vi "Thermistor Example.vi"() -> ()   [LabVIEW 2012]
doc: "An example that uses an Arduino to read the temperature from a thermistor. The user is able to select the supply voltage, paired resistance, analog input pin and units (C, F, K)."
uses:
  <vilib>/LabVIEW Interface for Arduino/Type Defs/Board Type.ctl
  <vilib>/LabVIEW Interface for Arduino/LabVIEW Interface for Arduino.lvlib
panel:
  in  "Paired Resistance (Ohms)":dbl=10000.0
  out "Temperature":dbl(slide) scale=0.0..100.0
  in  "Units":enum16{"Celsius", "Fahrenheit", "Kelvin"}(ring)
  in  "Thermistor AI Pin":u8=1
  in  "Stop":bool
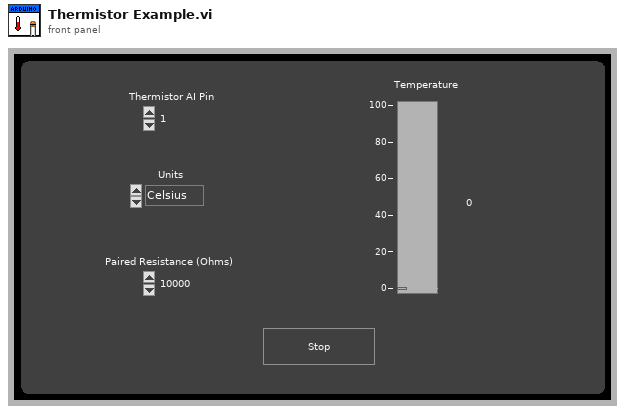
[diagram p1: front panel]
types:
  T1 = typedef "LabVIEW Interface for Arduino.lvlib/Board Type.ctl" = enum16{"Uno", "Dimuelanove w/Atmega 328", "Mega 2560"}
  T2 = typedef "LabVIEW Interface for Arduino.lvlib/Arduino Resource.ctl" = cluster{"VISA resource":refnum<visa-resource-name>, "Board Type":T1, "Connection Type":enum8{"USB / Serial"}, "Bytes Per Packet (15)":u8}
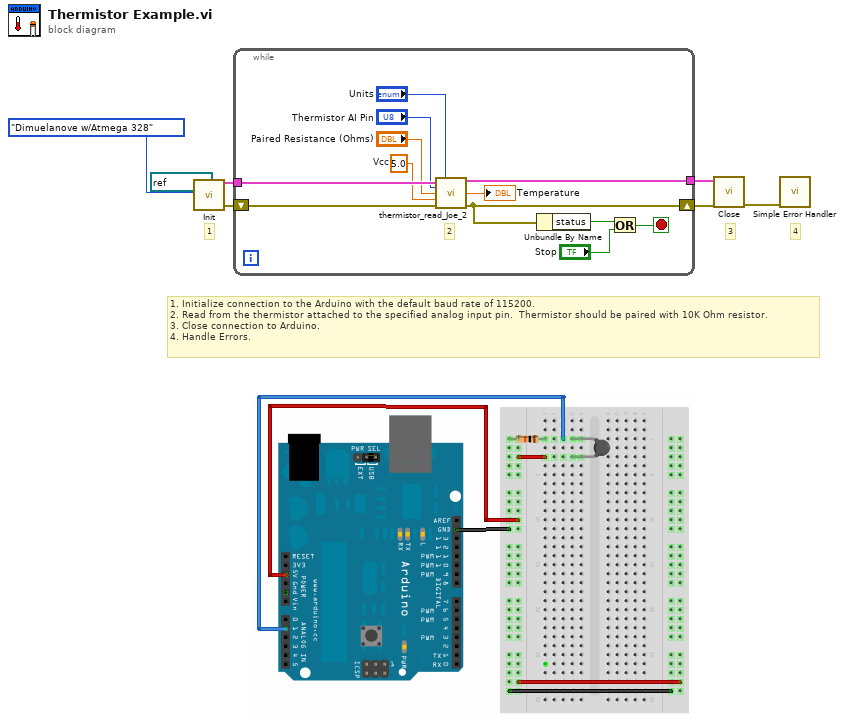
[diagram p0: block diagram]
diagram:
  # "4"
  # "3"
  # "1"
  # "1. Initialize connection to the Arduino with the default baud rate of 115200.\n2. Read from the thermistor attached to the specified analog input pin.  Thermistor should be paired with 10K Ohm resistor.\n3. Close connection to Arduino.\n4. Handle Errors."
  n1 = call <vilib>:"Init.vi"("VISA resource"=refnum<visa-resource-name> "COM4", "Board Type (Uno)"=Board_Type."Dimuelanove w/Atmega 328") -> ("Arduino Resource"=w7:T2, "error out"=w6:errorcluster)  [unwired: 16 in]
  n2 = while {
    tunnel: w7 -> [w16]
    shift-right: [w14] -> w4
    shift-left: w6 -> [w15]
    tunnel: [w13] -> w5
    stop <- w17 stop-if-true
    w11 = 5.0  # Vcc
    # "2"
    n3 = call "thermistor_read_Joe_2.vi"("Arduino Resource"=w16, "Units (C)"="Units", "Thermistor AI Pin (0)"="Thermistor AI Pin", "Paired Resistance (10K Ohms)"="Paired Resistance (Ohms)", "Vcc (5 v)"=w11, "error in"=w15) -> ("Arduino Resource"=w13:T2, "Temperature"=→"Temperature":dbl, "error out"=w14:errorcluster)  [unwired: 7 in]
    n4 = Unbundle By Name(w14) -> ("status"=w19:bool)
    n5 = Or(x=w19, y="Stop") -> (x .or. y?=w17:bool)
  }
  n6 = call <vilib>:"Close.vi"("Arduino Resource"=w5, "error in"=w4) -> ("error out"=w3:errorcluster)  [unwired: 13 in]
  n7 = call <vilib>:"Simple Error Handler.vi"("error in (no error)"=w3) -> ()  [unwired: 4 in, 5 out]
